vi "VariantToVoid.vi"(8 "error in (no error)":errorcluster, 11 "Void":variant) -> (0 "error out":errorcluster, 1 "DecomposedVariant":T1[](array[typedef]), 2 "Type":string, 3 "Value":string)   [LabVIEW 2019, in "BlueVariantView.lvlib"]
uses:
  BlueVariantView.lvlib
  DecomposedMap.ctl
  DecomposedVariant.ctl
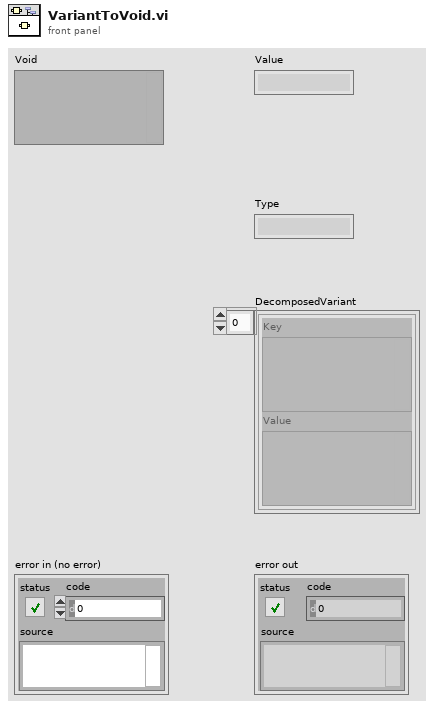
[diagram p1: front panel]
types:
  T1 = typedef "BlueVariantView.lvlib/DecomposedMap.ctl" = cluster{"Key":variant, "Value":variant}
  T2 = typedef "BlueVariantView.lvlib/DecomposedVariant.ctl" = cluster{"Key":string, "Value":variant}
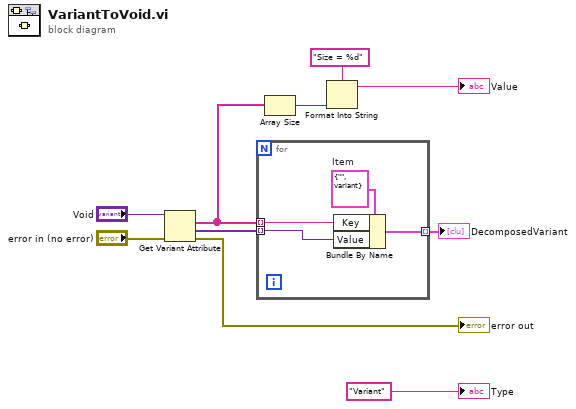
[diagram p0: block diagram]
diagram:
  n1 = Get Variant Attribute(Variant="Void", error in="error in (no error)") -> (names=w2:string[], values=w4:variant[], error out=→"error out":errorcluster)  [unwired: 2 in, 1 out]
  n2 = for {
    tunnel: [w14] -> w7 mode=indexing
    tunnel: w2 -> [w13] mode=indexing
    tunnel: w4 -> [w12] mode=indexing
    w11 = T2 {"Key"="", "Value"=variant}  # Item
    n3 = Bundle By Name(cluster=w11, "Key"=w13, "Value"=w12) -> (w14:T2)
  }
  "DecomposedVariant" <- w7
  n4 = Array Size(array=w2) -> (size(s)=w1:i32)
  n5 = Format Into String(format string="Size = %d", w1) -> (resulting string=→"Value":string)  [unwired: 2 in, 1 out]
  "Type" <- "Variant" ("Type")
